vi "Return Setpoint Status.vi"(4 "error":string, 6 "Status":T1, 8 "error in (no error)":errorcluster, 9 "Setpoint Name":string, 10 "IED Name":string, 11 "SCADA in":refnum<class "SCADA.lvclass">) -> (0 "error out":errorcluster, 3 "SCADA out":refnum<class "SCADA.lvclass">)   [LabVIEW 2015, in "SCADA Core.lvlib" / "SCADA.lvclass"]
uses:
  SCADA.lvclass
  SCADA Abstract Messages/IED Setpoint Status Msg/IED Setpoint Status.ctl
  SCADA.lvclass/SCADA.ctl
  <vilib>/ActorFramework/Actor/Actor.lvclass/Actor.ctl
  <vilib>/ActorFramework/Actor/Actor.lvclass
  SCADA Abstract Messages/IED Setpoint Status Msg/IED Setpoint Status Msg.lvclass
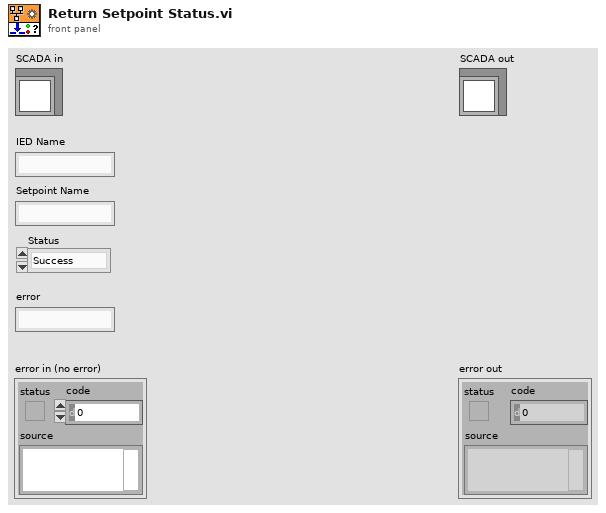
[diagram p1: front panel]
types:
  T1 = typedef "SCADA Core.lvlib/IED Setpoint Status Msg.lvclass/IED Setpoint Status.ctl" = enum16{"Success", "Failure", "Multiple Success", "Multiple Failure"}
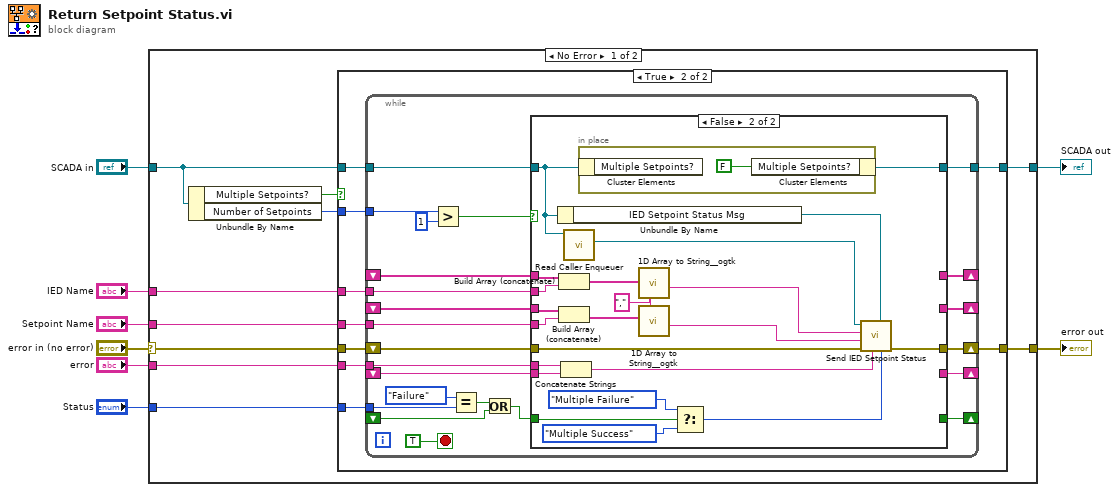
[diagram p0: block diagram]
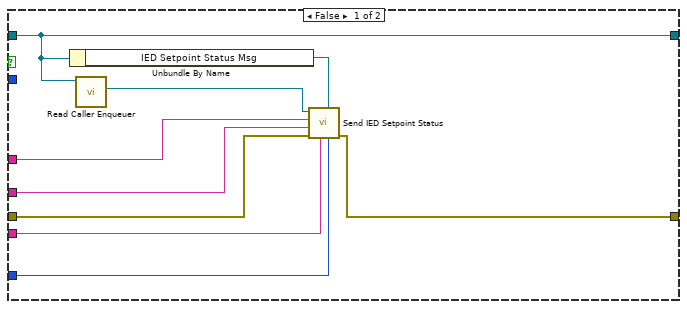
[diagram p2: hidden frame]
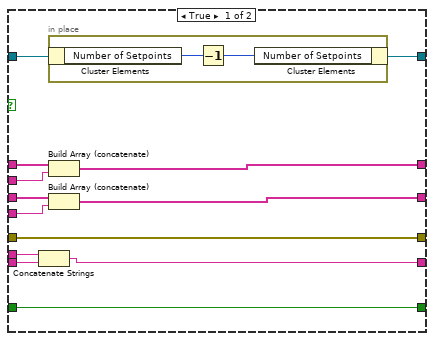
[diagram p3: hidden frame]
diagram:
  n1 = case shown="No Error" "error in (no error)" {
    selector: "error in (no error)" -> [w16 w99]
    tunnel: [w15 w99] -> w7
    tunnel: [w11 w98] -> w5
    tunnel: "SCADA in" -> [w12 w98]
    tunnel: "IED Name" -> [w18 _]
    tunnel: "Setpoint Name" -> [w17 _]
    tunnel: "error" -> [w14 _]
    tunnel: "Status" -> [w13 _]
    frame No Error {
      n2 = Unbundle By Name(w12) -> ("Multiple Setpoints?"=w10:bool, "Number of Setpoints"=w9:u8)
      n3 = case shown="True" w10 {
        tunnel: w18 -> [w25 w35]
        tunnel: w17 -> [w24 w34]
        tunnel: w16 -> [w23 w33]
        tunnel: [w22 w30] -> w15
        tunnel: w14 -> [w21 w32]
        tunnel: w13 -> [w20 w31]
        tunnel: w12 -> [w19 w36]
        tunnel: [w19 w29] -> w11
        tunnel: w9 -> [_ w28]
        frame False {
          n4 = Unbundle By Name(w19) -> ("IED Setpoint Status Msg"=w27:refnum<class "IED Setpoint Status Msg.lvclass">)
          n5 = call <vilib>:"Read Caller Enqueuer.vi"("Actor"=w19) -> ("Caller Enqueuer"=w26:refnum<class "Message Enqueuer.lvclass">)  [unwired: 10 in]
          n6 = call "Send IED Setpoint Status.vi"("Status"=w20, "IED Setpoint Status Msg"=w27, "Error String"=w21, "error in (no error)"=w23, "Setpoint Name"=w24, "IED Name"=w25, "Message Enqueuer in"=w26) -> ("error out"=w22:errorcluster)  [unwired: 3 in, 1 out]
        }
        frame True {
          n7 = while {
            tunnel: w36 -> [w42]
            tunnel: w35 -> [w45]
            tunnel: w34 -> [w48]
            tunnel: w32 -> [w52]
            tunnel: w31 -> [w54]
            shift-right: [w58] -> _
            shift-left: _ -> [w55]
            shift-right: [w51] -> _
            shift-left: _ -> [w50]
            shift-right: [w47] -> _
            shift-left: _ -> [w46]
            shift-right: [w44] -> _
            shift-left: _ -> [w43]
            shift-right: [w41] -> w30
            shift-left: w33 -> [w49]
            tunnel: [w40] -> w29
            tunnel: w28 -> [w38]
            stop <- TRUE stop-if-true
            n8 = Greater?(x=w38, y=u8 1) -> (0:w37:bool)
            n9 = Equal?(x=IED_Setpoint_Status."Failure" ("y"), y=w54) -> (x = y?=w57:bool)
            n10 = Or(x=w57, y=w55) -> (x .or. y?=w53:bool)
            n11 = case shown="False" w37 {
              tunnel: [w72 _] -> w58
              tunnel: w53 -> [w72 w94]
              tunnel: w52 -> [w71 w96]
              tunnel: [w70 _] -> w51
              tunnel: w50 -> [w69 w95]
              tunnel: w49 -> [w64 w89]
              tunnel: w48 -> [w60 w80]
              tunnel: [w68 _] -> w47
              tunnel: w46 -> [w67 w81]
              tunnel: w45 -> [w61 w82]
              tunnel: [w66 _] -> w44
              tunnel: w43 -> [w65 w83]
              tunnel: w42 -> [w63 w85]
              tunnel: [w64 w86] -> w41
              tunnel: [w62 w84] -> w40
              frame True {
                n12 = Concatenate Strings(w71, w69) -> (w70:string)
                n13 = in-place {
                  n14 = in-place-cluster #1(w63) -> ("Number of Setpoints"=w74:u8)
                  n15 = Decrement(x=w74) -> (x-1=w73:u8)
                  n16 = in-place-cluster #1("Number of Setpoints"=w73) -> (w62:refnum<class "SCADA.lvclass">)
                }
                n17 = Build Array (concatenate)(w65, w61) -> (w66:string[])
                n18 = Build Array (concatenate)(w67, w60) -> (w68:string[])
              }
              frame False {
                w77 = "," ("delimiter (Tab)")
                n19 = Unbundle By Name(w85) -> ("IED Setpoint Status Msg"=w91:refnum<class "IED Setpoint Status Msg.lvclass">)
                n20 = Build Array (concatenate)(w83, w82) -> (w79:string[])
                n21 = Build Array (concatenate)(w81, w80) -> (w78:string[])
                n22 = Concatenate Strings(w96, w95) -> (w87:string)
                n23 = call <vilib>:"Read Caller Enqueuer.vi"("Actor"=w85) -> ("Caller Enqueuer"=w90:refnum<class "Message Enqueuer.lvclass">)  [unwired: 10 in]
                n24 = in-place {
                  n25 = in-place-cluster #2(w85) -> ()  [unwired: 1 out]
                  n26 = in-place-cluster #2("Multiple Setpoints?"=FALSE) -> (w84:refnum<class "SCADA.lvclass">)
                }
                n27 = call <userlib>:"1D Array to String__ogtk.vi"("delimiter (Tab)"=w77, "Array of Strings"=w79) -> ("delimited string"=w75:string)  [unwired: 9 in]
                n28 = call <userlib>:"1D Array to String__ogtk.vi"("delimiter (Tab)"=w77, "Array of Strings"=w78) -> ("delimited string"=w76:string)  [unwired: 9 in]
                n29 = Select(t=IED_Setpoint_Status."Multiple Failure" ("y"), s=w94, f=IED_Setpoint_Status."Multiple Success" ("y")) -> (s? t:f=w88:T1)
                n30 = call "Send IED Setpoint Status.vi"("Status"=w88, "IED Setpoint Status Msg"=w91, "Error String"=w87, "error in (no error)"=w89, "Setpoint Name"=w76, "IED Name"=w75, "Message Enqueuer in"=w90) -> ("error out"=w86:errorcluster)  [unwired: 3 in, 1 out]
              }
            }
          }
        }
      }
    }
    frame Error {
    }
  }
  "error out" <- w7
  "SCADA out" <- w5
